vi "Get_xcursors_from_graph.vi"(11 "WaveformGraph in":refnum<vi>) -> (3 "Array":dbl[](array[numeric]))   [LabVIEW 2015]
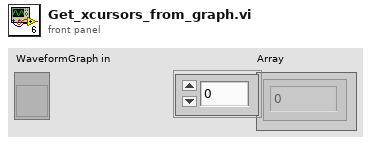
[diagram p1: front panel]
types:
  T1 = typedef "LVCursorListTypeDef.ctl" = cluster{"Name":string, "Color":u32, "Style":u8, "Point Style":u8, "Name Visible":bool, "Allow Drag":bool, "Cursor Mode":u32, "Plot":i32, "Index":i32, "Position":cluster{"X":dbl, "Y":dbl}, "X Scale":u32, "Y Scale":u32, "Watch Plots":i32[], "Watch All Plots":bool, "Plot Area":i32, "Label Offset":cluster{"X":dbl, "Y":dbl}}[]
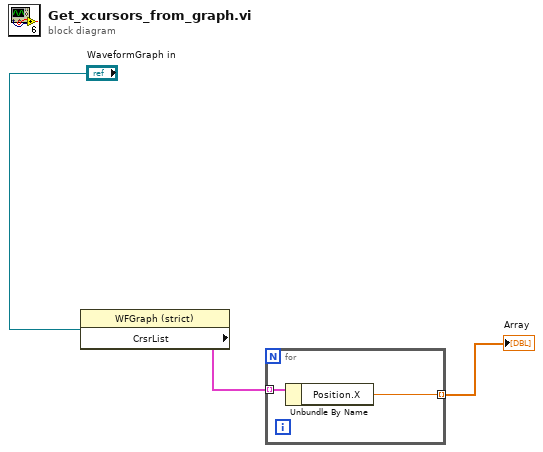
[diagram p0: block diagram]
diagram:
  n1 = property class="WFGraph (strict)"(reference="WaveformGraph in") -> ("CrsrList"=w1:T1)  [unwired: 1 in, 2 out]
  n2 = for {
    tunnel: w1 -> [w5] mode=indexing
    tunnel: [w4] -> w3 mode=indexing
    n3 = Unbundle By Name(w5) -> ("Position.X"=w4:dbl)
  }
  "Array" <- w3
